vi "Draw++.vi"(1 "Width":i32=25, 2 "PosArray":cluster{"P_X":i32, "P_Y":i32}[](array[cluster]), 3 "Color":u32(colorbox)=16711680, 4 "Image In":T1) -> (0 "Image In 2":T1)   [LabVIEW 2014]
uses:
  <vilib>/vision/Image Controls.llb/IMAQ Image.ctl
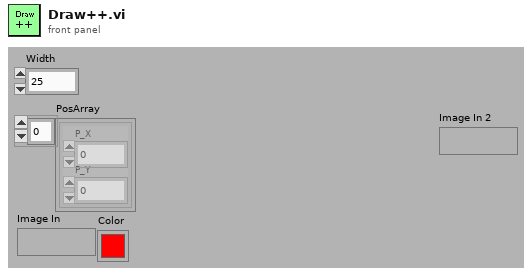
[diagram p1: front panel]
types:
  T1 = typedef "IMAQ Image.ctl" = refnum<image>
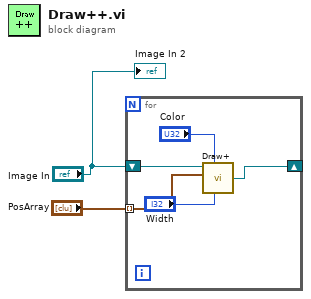
[diagram p0: block diagram]
diagram:
  n1 = for {
    tunnel: "PosArray" -> [w7] mode=indexing
    shift-right: [w5] -> _
    shift-left: "Image In" -> [w6]
    n2 = call "Draw+.vi"("Width"="Width", "Color"="Color", "input cluster"=w7, "Image In"=w6) -> ("Image Out"=w5:T1)  [unwired: 2 in]
  }
  "Image In 2" <- "Image In"
